vi "PriorRecord.vi"(0 "reference in":refnum<class "CustomersData.lvclass">, 5 "error in (no error)":errorcluster) -> (14 "reference out":refnum<class "CustomersData.lvclass">, 19 "error out":errorcluster)   [LabVIEW 2020, in "CustomersData.lvclass"]
uses:
  CustomersData.lvclass
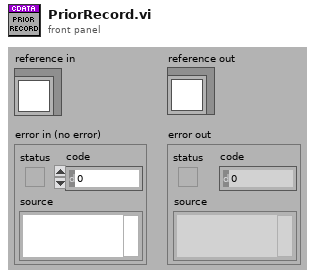
[diagram p1: front panel]
types:
  T1 = typedef "CustomersData.lvclass/ObjectAttributes.ctl" = cluster{"_customers":string[], "_current":i32}
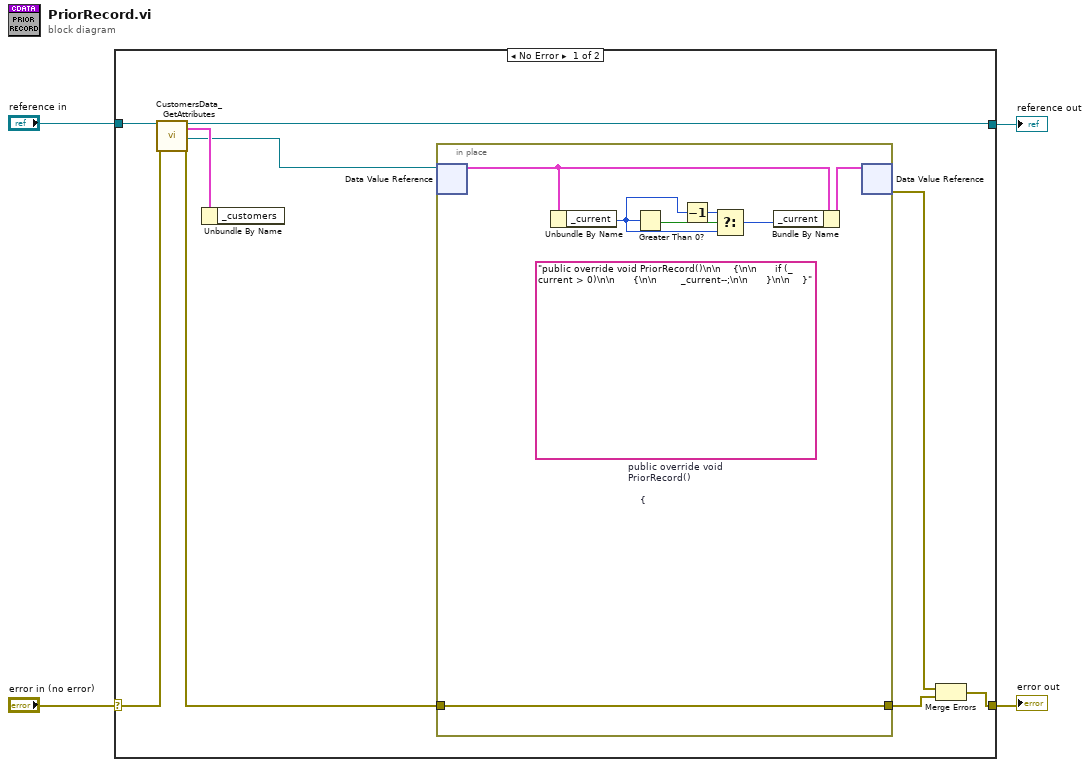
[diagram p0: block diagram]
diagram:
  n1 = case shown="No Error" "error in (no error)" {
    selector: "error in (no error)" -> [w12 w22]
    tunnel: [w9 w22] -> w3
    tunnel: [w8 w21] -> w1
    tunnel: "reference in" -> [w13 w21]
    frame No Error {
      n2 = call "CustomersData_GetAttributes.vi"("reference in"=w13, "error in (no error)"=w12) -> ("reference out"=w8:refnum<class "CustomersData.lvclass">, "Data"=w11:T1, "DataRef"=w7:refnum<data-value>, "error out"=w6:errorcluster)  [unwired: 14 in]
      n3 = Unbundle By Name(w11) -> ()  [unwired: 1 out]
      n4 = in-place {
        in-place-border: w6 -> [w19]
        in-place-border: [w19] -> w5
        (unwired) "public override void PriorRecord()\n\n    {\n\n      if (_current > 0)\n\n      {\n\n        _current--;\n\n      }\n\n    }"  # public override void PriorRecord()      {        if (_current > 0)        {          _current--;        }      }
        n5 = in-place-dvr #1(w7) -> (w18:T1)  [unwired: 1 out]
        n6 = Unbundle By Name(w18) -> ("_current"=w16:i32)
        n7 = Greater Than 0?(x=w16) -> (x > 0?=w17:bool)
        n8 = Decrement(x=w16) -> (x-1=w14:i32)
        n9 = Select(t=w14, s=w17, f=w16) -> (s? t:f=w15:i32)
        n10 = Bundle By Name(cluster=w18, "_current"=w15) -> (w20:T1)
        n11 = in-place-dvr #1(w20) -> (w10:errorcluster)  [unwired: 1 out]
      }
      n12 = Merge Errors(w10, w5) -> (w9:errorcluster)
    }
    frame Error {
    }
  }
  "error out" <- w3
  "reference out" <- w1
